vi "Transport To Actor Type.vi"(10 "Spawn":refnum<class "Spawn.lvclass">) -> (2 "Actor Type":T1)   [LabVIEW 2025, in "jettl.lvlib"]
uses:
  jettl.lvlib
  Actor Type.ctl
  Spawn/Spawn/Spawn.lvclass
  Transport/Transport/Transport.lvclass
  Transport/Queue/Queue.lvlib
  Transport/Event/Event.lvlib
  Transport/Notifier/Notifier.lvlib
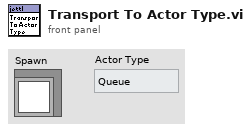
[diagram p1: front panel]
types:
  T1 = typedef "jettl.lvlib/Actor Type.ctl" = enum16{"Queue", "Event", "Notifier"}
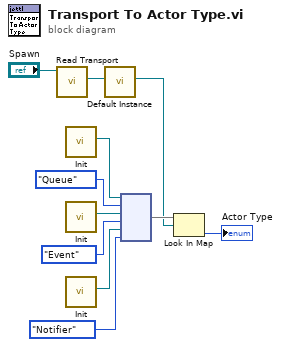
[diagram p0: block diagram]
diagram:
  n1 = call-dynamic "Read Transport.vi"("Spawn in"="Spawn") -> ("Transport"=w2:refnum<class "Transport.lvclass">)  [unwired: 10 in]
  n2 = call "Init.vi"() -> ("Transport"=w11:refnum<class "Transport.lvclass">)  [unwired: 11 in]
  n3 = call "Init.vi"() -> ("Transport"=w9:refnum<class "Transport.lvclass">)  [unwired: 11 in]
  n4 = call "Init.vi"() -> ("Transport"=w8:refnum<class "Transport.lvclass">)  [unwired: 11 in]
  n5 = call "Default Instance.vi"("Instance"=w2) -> ("Default Instance"=w1:refnum<class "Transport.lvclass">)  [unwired: 10 in]
  n6 = node(w11, Actor_Type."Queue" ("Actor Type"), w9, Actor_Type."Event" ("Actor Type"), w8, Actor_Type."Notifier" ("Actor Type")) -> (w5:map{refnum<class "Transport.lvclass">, T1})
  n7 = Look In Map(map=w5, key=w1) -> (value=→"Actor Type":T1)  [unwired: 1 in, 1 out]
